vi "chooseCase.vi"(9 "Robot":refnum<class "Robot.lvclass">, 10 "Game in":refnum<class "Game.lvclass">, 11 "Utilities in":refnum<class "Utilities.lvclass">) -> (3 "States":enum16{"PassObserver", "Halt", "Exit"}(ring))   [LabVIEW 2023, in "PassObserverTactic.lvclass"]
uses:
  PassObserverTactic.lvclass
  Robot_class/Robot.lvclass
  Game_class/Game.lvclass
  Utilities_class/Utilities.lvclass
  Game_class/Game.lvclass/Game.ctl
  Team_class/Team.lvclass/Team.ctl
  Robot_class/roles.ctl
  Object_class/Object.lvclass/Object.ctl
  Parameters_class/Parameters.lvclass/Parameters.ctl
  Robot_class/Robot.lvclass/Robot.ctl
  Object_class/Read x.vi
  Object_class/Read y.vi
  Game_class/Read OffensiveTeam.vi
  Game_class/Read BallRef.vi
  Game_class/Read Parameters.lvclass.vi
  Game_class/Read FieldRef.vi
  Parameters_class/Read AttakingOurselves.vi
  Team_class/Read OffensivePlay.vi
  Team_class/Read RobotRef.vi
  Robot_class/Read tactic.vi
  Robot_class/Read dest_orientation.vi
  Ball_class/Ball.lvclass
  Ally_class/Ally.lvclass
  Parameters_class/Parameters.lvclass
  Field_class/Field.lvclass
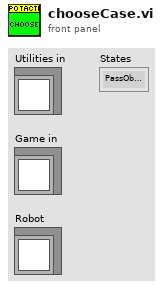
[diagram p1: front panel]
types:
  T1 = typedef "OffensivePlay.ctl" = enum16{"TableWithStriker", "TableWith2ndStrikerPlay", "PrepareDoublePass", "PrepareRollToPass", "SimplePass", "PreparePass", "PassToStriker", "BallOutOfField", "PassTo2ndStriker", "StopOffensive", "Prepare Penalty Enemy", "EnemyPossessionAtEnemyField", "EnemyPossesionAtOurField", "TestPlay", "PreparePenaltyAlly", "KickPenaltyAlly", "PrepareKickoffAlly", "PrepareKickoffEnemy", "IndirectEnemy", "DirectEnemy", "NormalGame", "DirectKick", "Pass", "Halt", "Timeout", "PassPlay", "PenaltyEnemy"}
  T2 = typedef "roles.ctl" = enum16{"BallChallengerAttackerVSS", "NormalAttackerVSS", "AttackerAimGoalVSS", "DefenderAreaVSS", "KeeperVSS", "Tabler", "TableFinalizer", "PrepareRollToPassRoller", "PrepareRollToPassReceiver", "SimplePassRoll", "SimplePassRollReceiver", "PenaltyDefense", "PreparePassReceiver 2", "PreparePassReceiver 1", "PassObserver", "Timeout", "Goto", "ZigZag", "None", "BallOutOfField", "DefenderArea", "Duelist", "AttackerStop", "FollowAttacker", "KeeperRole", "KickPenalty", "AttackerAimGoal", "AttackerBlock", "Marker", "Halt", "Shoot", "PassKicker", "PassReceiver", "TestRole", "PenaltyAttacker"}
  T3 = typedef "tactics.ctl" = enum16{"ReceivePassInFuturePoint", "Roller", "PrepareRollToPassRollerGoTo", "PrepareRollToPassReceiverGoTo", "WaitRoll", "PositionToRoll", "PenaltyAttacker", "PassObserver", "PenaltyDefense", "TableReceiverTactic", "Test", "DefendGoal", "Marker", "FollowAttacker", "DefendArea", "Shoot", "AttackerAimGoal", "AttackerBallOutOfField", "AttackerBlock", "AttackerStop", "Duelist", "Halt", "ZigZag", "GoTo", "Timeout", "KickToPassReceiver", "PositionToReceivePass", "DefendAreaVSS", "DefendGoalVSS", "KickVSS", "AttackVSS", "DispBallVSS", "PenaltyAttackVSS", "WaitPass"}
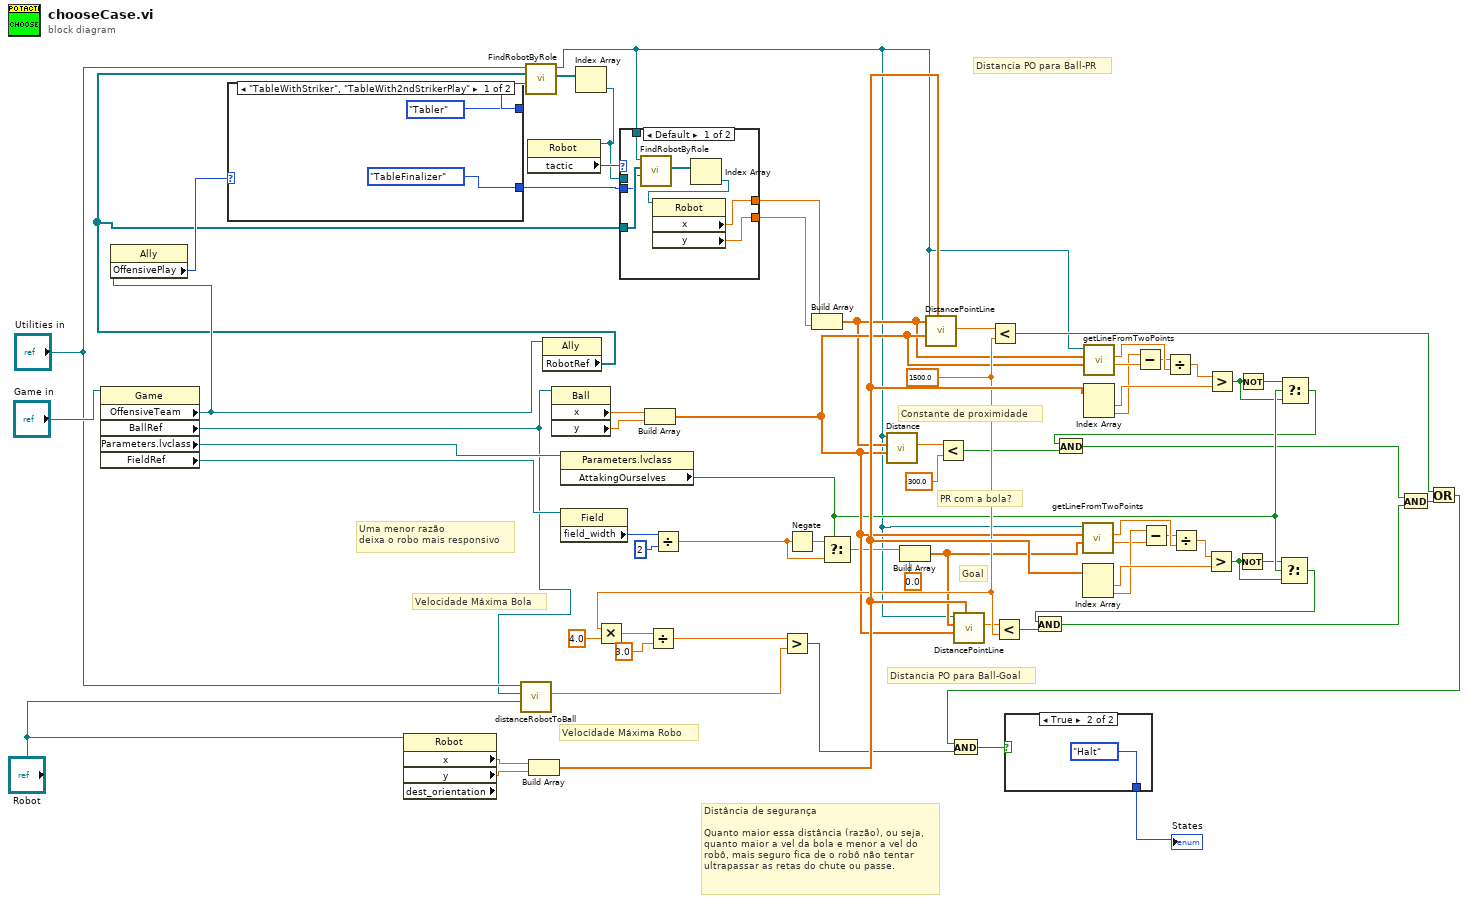
[diagram p0: block diagram]
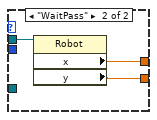
[diagram p2: hidden frame]
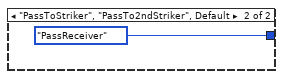
[diagram p3: hidden frame]
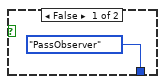
[diagram p4: hidden frame]
diagram:
  w57 = 1500.0 ("y")
  # "Uma menor razão\ndeixa o robo mais responsivo"
  # "PR com a bola?"
  # "Constante de proximidade"
  # "Distancia PO para Ball-Goal"
  # "Distancia PO para Ball-PR"
  # "Goal"
  # "Distância de segurança\n\nQuanto maior essa distância (razão), ou seja,\nquanto maior a vel da bola e menor a vel do\nrobô, mais seguro fica de o robô não tentar\nultrapassar as retas do chute ou passe."
  # "Velocidade Máxima Robo"
  # "Velocidade Máxima Bola"
  n1 = property class="Game"(reference="Game in") -> ("OffensiveTeam"=w9:refnum<class "Ally.lvclass">, "BallRef"=w10:refnum<class "Ball.lvclass">, "Parameters.lvclass"=w16:refnum<class "Parameters.lvclass">, "FieldRef"=w32:refnum<class "Field.lvclass">)  [unwired: 1 in, 2 out]
  n2 = property class="Ally"(reference=w9) -> ("OffensivePlay"=w8:T1)  [unwired: 1 in, 2 out]
  n3 = case shown="\"TableWithStriker\", \"TableWith2ndStrikerPlay\"" w8 {
    tunnel: [roles."Tabler" ("role") roles."PassReceiver" ("role")] -> w12
    tunnel: [roles."TableFinalizer" ("role") _] -> w2
    frame "TableWithStriker", "TableWith2ndStrikerPlay" {
    }
    frame "PassToStriker", "PassTo2ndStriker", Default {
    }
  }
  n4 = property class="Robot" props=["x", "y", "dest_orientation"](reference="Robot") -> ("x"=w18:dbl, "y"=w14:dbl)  [unwired: 1 in, 3 out]
  n5 = call "distanceRobotToBall.vi"("Robot"="Robot", "Ball"=w10, "Utilities in"="Utilities in") -> ("Distance Robot To Ball"=w28:dbl)  [unwired: 6 in, 2 out]
  n6 = Build Array(w18, w14) -> (w58:dbl[])
  n7 = property class="Ally"(reference=w9) -> ("RobotRef"=w3:refnum<class "Robot.lvclass">[])  [unwired: 1 in, 2 out]
  n8 = call "FindRobotByRole.vi"("role"=w12, "RobotRef"=w3, "Utilities in"="Utilities in") -> ("Robots"=w13:refnum<class "Robot.lvclass">[], "Utilities out"=w1:refnum<class "Utilities.lvclass">)  [unwired: 6 in, 1 out]
  n9 = property class="Ball"(reference=w10) -> ("x"=w19:dbl, "y"=w17:dbl)  [unwired: 1 in, 2 out]
  n10 = property class="Parameters.lvclass"(reference=w16) -> ("AttakingOurselves"=w53:bool)  [unwired: 1 in, 2 out]
  n11 = property class="Field"(reference=w32) -> ("field_width"=w33:i32)  [unwired: 1 in, 2 out]
  n12 = Index Array(array=w13) -> (element=w6:refnum<class "Robot.lvclass">)  [unwired: 1 in]
  n13 = property class="Robot"(reference=w6) -> ("tactic"=w7:T3)  [unwired: 1 in, 2 out]
  n14 = Multiply(x=w57, y=4.0) -> (x*y=w24:dbl)
  n15 = case shown="Default" w7 {
    tunnel: w6 -> [_ w83]
    tunnel: [w75 w82] -> w5
    tunnel: [w74 w81] -> w4
    tunnel: w3 -> [w80 _]
    tunnel: w2 -> [w79 _]
    tunnel: w1 -> [w78 _]
    frame Default {
      n16 = call "FindRobotByRole.vi"("role"=w79, "RobotRef"=w80, "Utilities in"=w78) -> ("Robots"=w77:refnum<class "Robot.lvclass">[])  [unwired: 6 in, 2 out]
      n17 = Index Array(array=w77) -> (element=w76:refnum<class "Robot.lvclass">)  [unwired: 1 in]
      n18 = property class="Robot"(reference=w76) -> ("x"=w75:dbl, "y"=w74:dbl)  [unwired: 1 in, 2 out]
    }
    frame "WaitPass" {
      n19 = property class="Robot"(reference=w83) -> ("x"=w82:dbl, "y"=w81:dbl)  [unwired: 1 in, 2 out]
    }
  }
  n20 = Build Array(w19, w17) -> (w56:dbl[])
  n21 = Divide(x=w24, y=3.0) -> (x/y=w26:dbl)
  n22 = Divide(x=w33, y=2) -> (x/y=w36:dbl)
  n23 = Greater?(x=w26, y=w28) -> (0:w27:bool)
  n24 = Negate(x=w36) -> (-x=w35:dbl)
  n25 = Build Array(w5, w4) -> (w47:dbl[])
  n26 = Select(t=w35, s=w53, f=w36) -> (s? t:f=w37:dbl)
  n27 = call-dynamic "Distance.vi"("P1"=w56, "P2"=w47, "Utilities in"=w1) -> ("Distance"=w30:dbl)  [unwired: 6 in, 2 out]
  n28 = Build Array(w37, 0.0 ("element")) -> (w55:dbl[])
  n29 = call-dynamic "DistancePointLine.vi"("Q"=w58, "P2"=w56, "P1"=w47, "Utilities in"=w1) -> ("distance"=w15:dbl)  [unwired: 5 in, 2 out]
  n30 = Less?(x=w30, y=300.0) -> (x < y?=w46:bool)
  n31 = call-dynamic "DistancePointLine.vi"("Q"=w58, "P2"=w56, "P1"=w55, "Utilities in"=w1) -> ("distance"=w39:dbl)  [unwired: 5 in, 2 out]
  n32 = Less?(x=w15, y=w57) -> (x < y?=w41:bool)
  n33 = Less?(x=w39, y=w57) -> (x < y?=w43:bool)
  n34 = call "getLineFromTwoPoints.vi"("Point 2"=w55, "Point 1"=w56, "Utilities in"=w1) -> ("linear coef"=w67:dbl, "angular coef"=w69:dbl)  [unwired: 4 in, 3 out]
  n35 = Index Array(array=w58) -> (element #1=w70:dbl, element #2=w68:dbl)  [unwired: 2 in]
  n36 = call "getLineFromTwoPoints.vi"("Point 2"=w56, "Point 1"=w47, "Utilities in"=w1) -> ("linear coef"=w60:dbl, "angular coef"=w62:dbl)  [unwired: 4 in, 3 out]
  n37 = Index Array(array=w58) -> (element #1=w64:dbl, element #2=w59:dbl)  [unwired: 2 in]
  n38 = Subtract(x=w59, y=w60) -> (x-y=w61:dbl)
  n39 = Subtract(x=w68, y=w67) -> (x-y=w65:dbl)
  n40 = Divide(x=w61, y=w62) -> (x/y=w63:dbl)
  n41 = Divide(x=w65, y=w69) -> (x/y=w66:dbl)
  n42 = Greater?(x=w66, y=w70) -> (0:w52:bool)
  n43 = Greater?(x=w63, y=w64) -> (0:w49:bool)
  n44 = Not(x=w52) -> (.not. x?=w51:bool)
  n45 = Not(x=w49) -> (.not. x?=w48:bool)
  n46 = Select(t=w51, s=w53, f=w52) -> (s? t:f=w54:bool)
  n47 = And(x=w54, y=w43) -> (x .and. y?=w45:bool)
  n48 = Select(t=w48, s=w53, f=w49) -> (s? t:f=w50:bool)
  n49 = And(x=w50, y=w46) -> (x .and. y?=w44:bool)
  n50 = And(x=w44, y=w45) -> (x .and. y?=w40:bool)
  n51 = Or(x=w41, y=w40) -> (x .or. y?=w42:bool)
  n52 = And(x=w42, y=w27) -> (x .and. y?=w29:bool)
  n53 = case shown="True" w29 {
    tunnel: [enum16{"PassObserver", "Halt", "Exit"}."PassObserver" ("States") enum16{"PassObserver", "Halt", "Exit"}."Halt" ("States")] -> w11
    frame False {
    }
    frame True {
    }
  }
  "States" <- w11
